vi "CoMP-S New AISAS Motors Check.vi"(8 "error in (no error)":errorcluster, 11 "Motor selection":enum32{"Rotation", "Difuser ", "Objective Lens"}(ring)=enum."Difuser ") -> (0 "error out":errorcluster)   [LabVIEW 2014]
uses:
  Controls/Global demo.vi
panel:
  out "element":u8
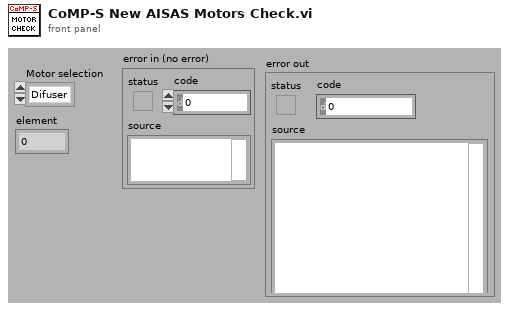
[diagram p1: front panel]
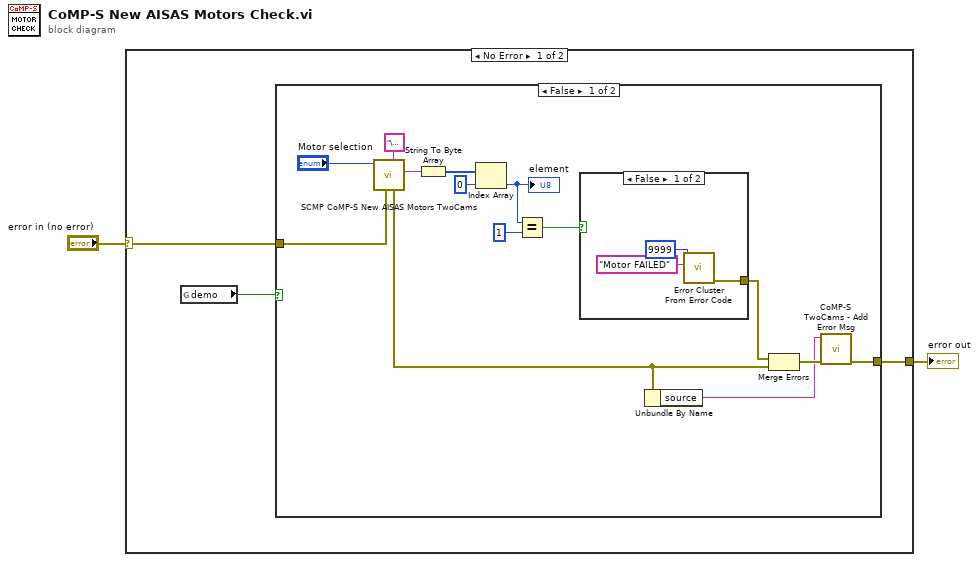
[diagram p0: block diagram]
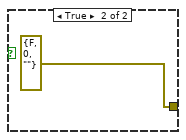
[diagram p2: hidden frame]
diagram:
  n1 = case shown="No Error" "error in (no error)" {
    selector: "error in (no error)" -> [w5 w25]
    tunnel: [w4 w25] -> w1
    frame No Error {
      n2 = global read "Global demo.vi" "demo"() -> (w3:bool)
      n3 = case shown="False" w3 {
        tunnel: w5 -> [w11 w24]
        tunnel: [w7 w24] -> w4
        frame False {
          n4 = call "SCMP CoMP-S New AISAS Motors TwoCams.vi"("Motion Code"="\u0004", "error in (no error)"=w11, "Motor selection"="Motor selection") -> ("Read Buffer Out"=w17:string, "error out"=w9:errorcluster)  [unwired: 5 in, 2 out]
          n5 = String To Byte Array(string=w17) -> (unsigned byte array=w16:u8[])
          n6 = Index Array(array=w16, index=0) -> (element=w14:u8)
          "element" <- w14
          n7 = Equal?(x=w14, y=u8 1) -> (x = y?=w12:bool)
          n8 = case shown="False" w12 {
            tunnel: [w22 errorcluster {"status"=FALSE, "code"=0, "source"=""} ("error in (no error) 2")] -> w10
            frame False {
              n9 = call <vilib>:"Error Cluster From Error Code.vi"("error message (\"\")"="Motor FAILED" ("error message (\"\")"), "error code (0)"=9999) -> ("error out"=w22:errorcluster)  [unwired: 7 in]
            }
            frame True {
            }
          }
          n10 = Unbundle By Name(w9) -> ("source"=w6:string)
          n11 = Merge Errors(w10, w9) -> (w8:errorcluster)
          n12 = call "CoMP-S TwoCams - Add Error Msg.vi"("error in"=w8, "error message (\"\")"=w6) -> ("errorout"=w7:errorcluster)  [unwired: 9 in]
        }
        frame True {
        }
      }
    }
    frame Error {
    }
  }
  "error out" <- w1
